vi "影像辨識-2.vi"() -> ()   [LabVIEW 2014]
uses:
  <vilib>/vision/NI_Vision_Development_Module.lvlib
panel:
  out "Image Pixels (U32) 3":u32[][](array[numeric])
  out "Image Pixels (U32) 2":u32[][](array[numeric])
  out "Image Pixels (U32)":u32[][](array[numeric])
  out "Pixel Value (U8)":u8
  out "Pixel Value (U32)":u32
  out "lumi 2":T1(plugin-control)
  out "saturastion":T1(plugin-control)
  in  "Stop (F)":bool
  out "Image Out":T1(plugin-control)
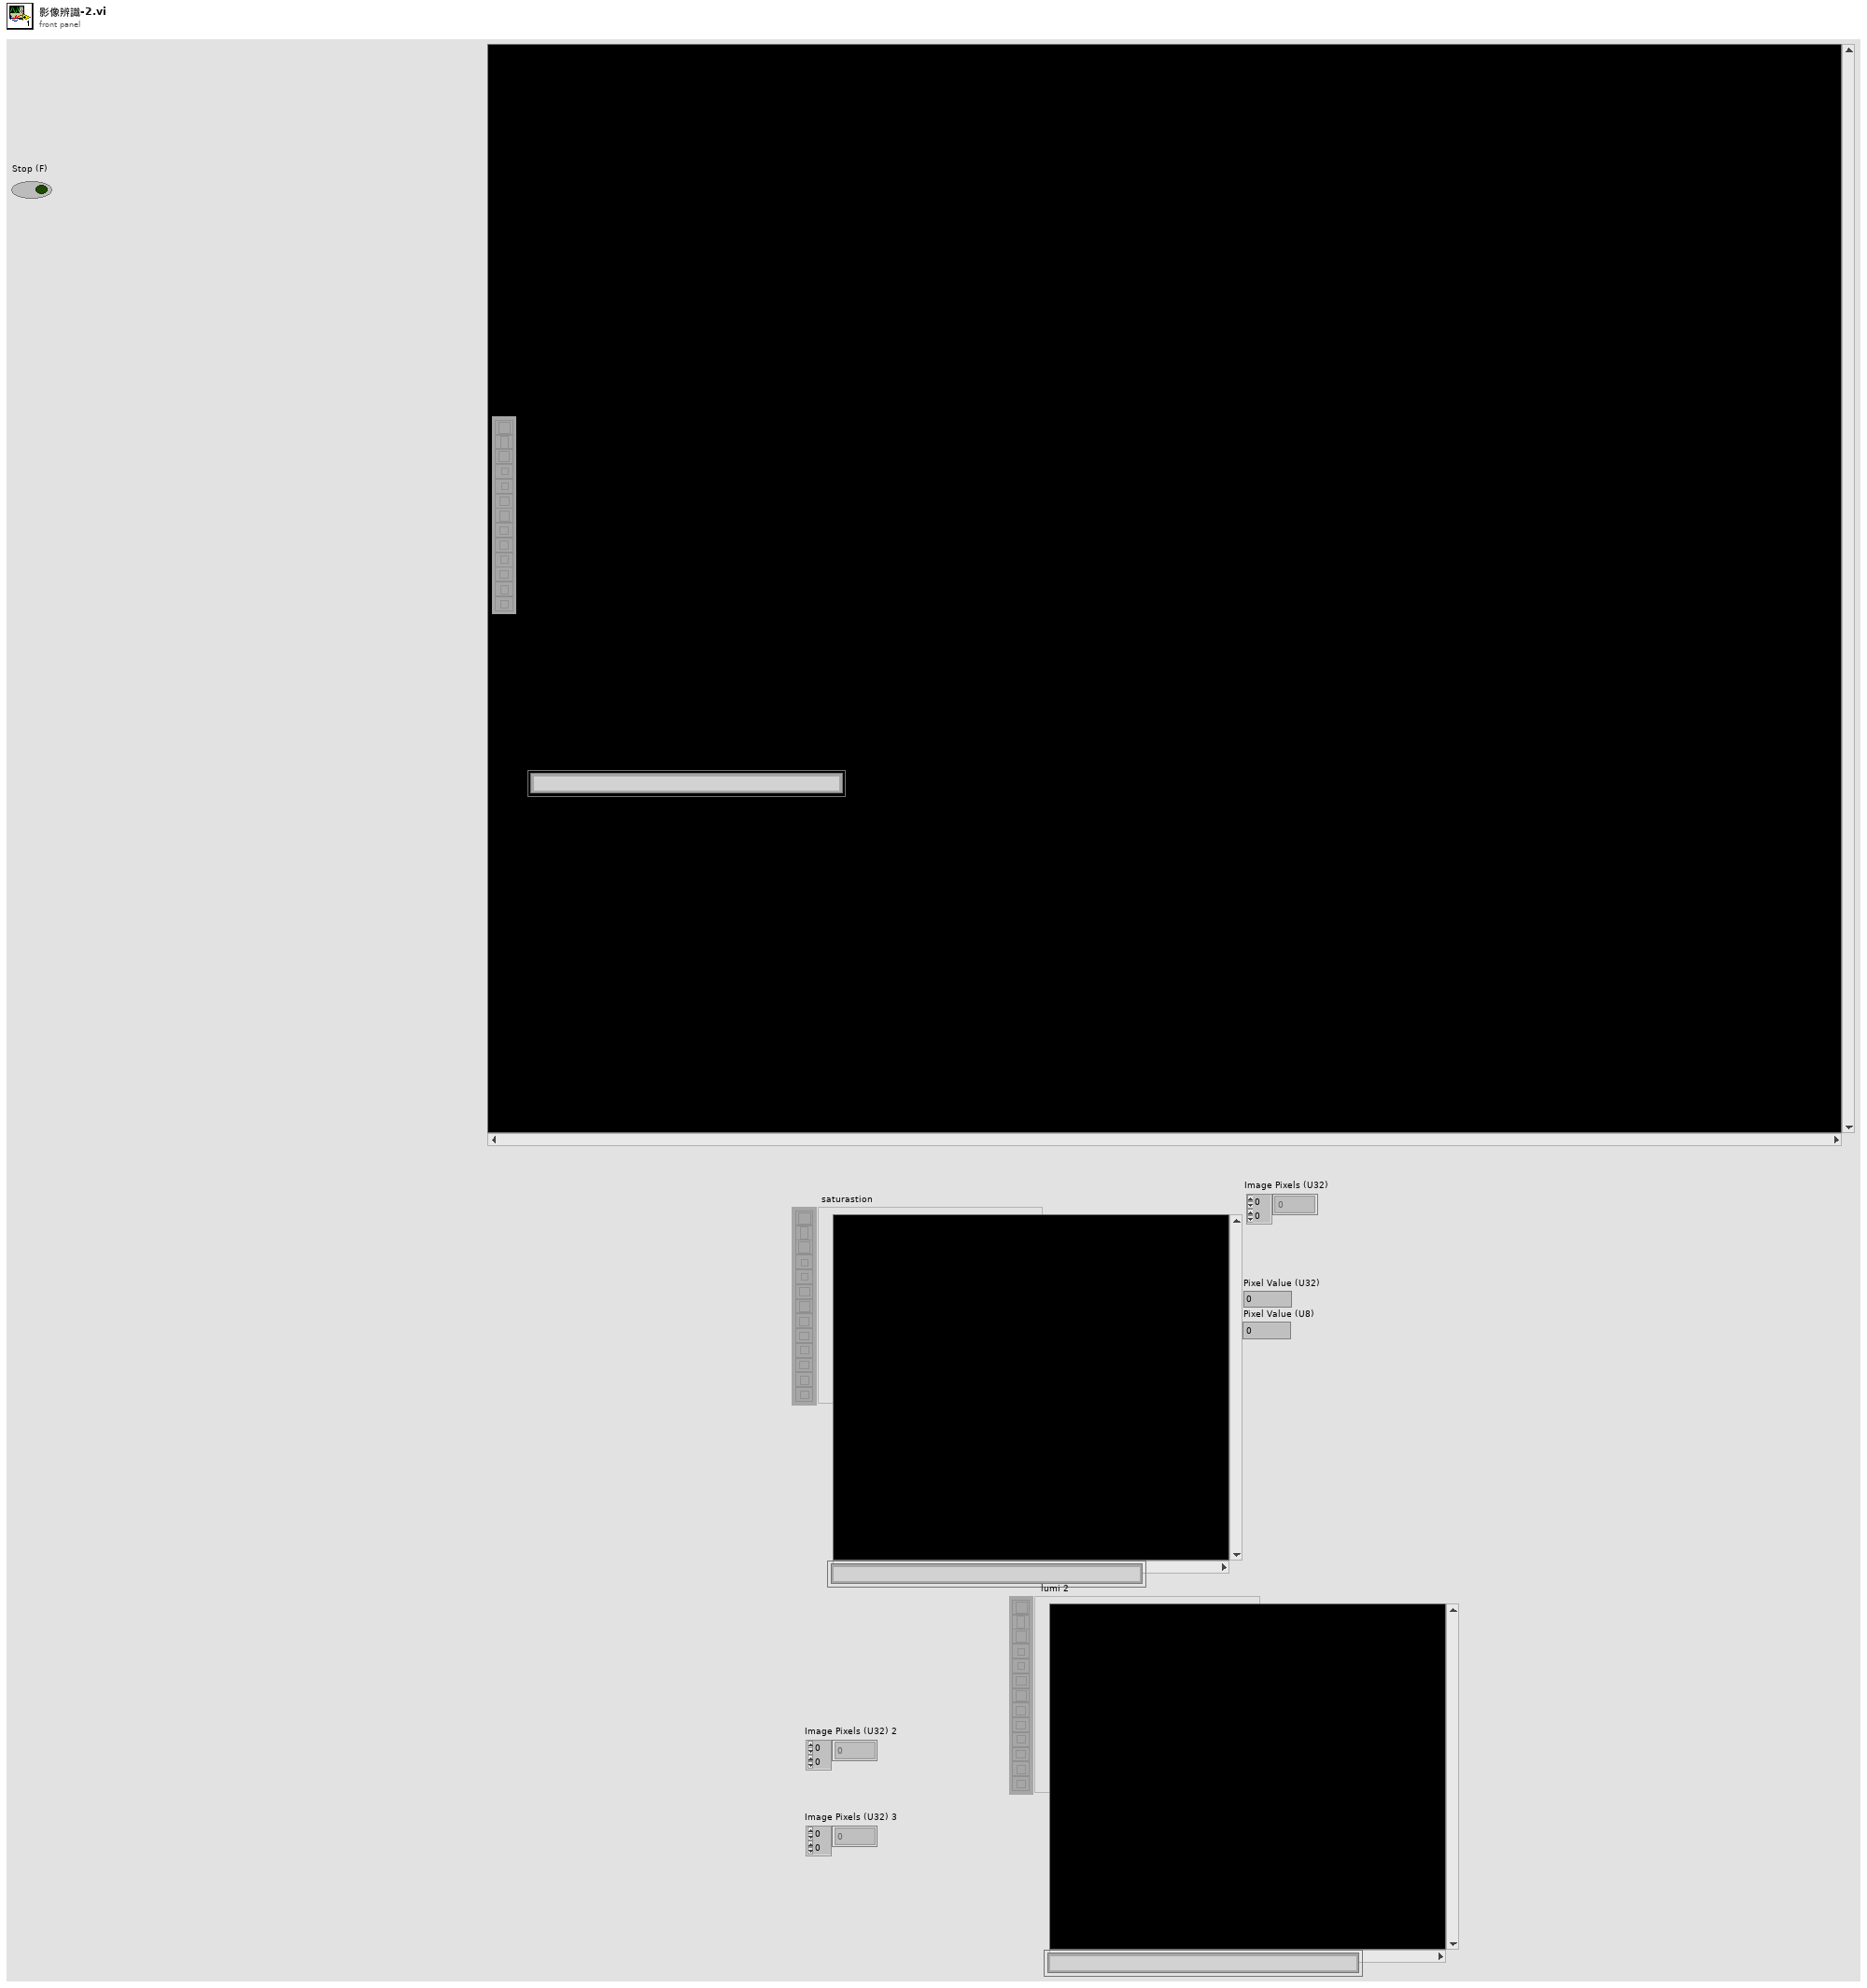
[diagram p1: front panel]
types:
  T1 = typedef "IMAQ Image.ctl" = refnum<image>
  T2 = typedef "Image Type" = u32
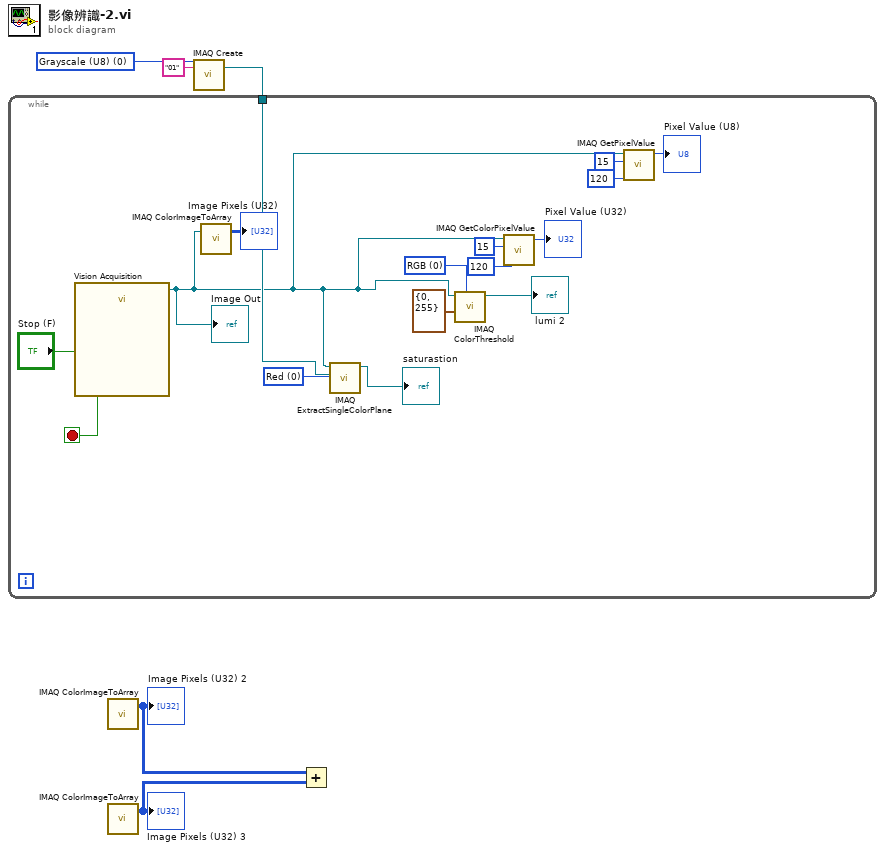
[diagram p0: block diagram]
diagram:
  w3 = T2 0 items=["Grayscale (U8)", "Grayscale (I16)", "Grayscale (SGL)", "Complex (CSG)", "RGB (U32)", "HSL (U32)", "RGB (U64)", "Grayscale (U16)"] ("Image Type")
  n1 = call "IMAQ ColorImageToArray"() -> ("Image Pixels (U32)"=w2:u32[][])  [unwired: 4 in, 2 out]
  "Image Pixels (U32) 2" <- w2
  n2 = call "IMAQ ColorImageToArray"() -> ("Image Pixels (U32)"=w1:u32[][])  [unwired: 4 in, 2 out]
  "Image Pixels (U32) 3" <- w1
  n3 = call "IMAQ Create"("Image Name"="01", "Image Type"=w3) -> ("New Image"=w5:T1)  [unwired: 3 in, 1 out]
  n4 = while {
    tunnel: w5 -> [w17]
    stop <- w20 stop-if-true
    w16 = u16 0 items=["RGB", "HSL", "HSV", "HSI"] ("Color Mode")
    w19 = 0 items=["Red", "Green", "Blue", "Hue", "Saturation", "Luminance", "Value", "Intensity"] ("Color Plane")
    n5 = call "Vision Acquisition"("Stop (F)"="Stop (F)") -> ("Image Out"=w7:T1, "Stopped"=w20:bool)  [unwired: 24 in, 1 out]
    "Image Out" <- w7
    n6 = call "IMAQ ColorImageToArray"("Image"=w7) -> ("Image Pixels (U32)"=→"Image Pixels (U32)":u32[][])  [unwired: 3 in, 2 out]
    n7 = call "IMAQ ExtractSingleColorPlane"("Color Plane"=w19, "Image Dst"=w17, "Image Src"=w7) -> ("Image Dst Out"=→"saturastion":T1)  [unwired: 7 in, 1 out]
    n8 = call "IMAQ ColorThreshold"("Color Mode"=w16, "Red or Hue Range"=cluster{"Lower value":i32, "Upper value":i32} {"Lower value"=0, "Upper value"=255}, "Image Src"=w7) -> ("Image Dst Out"=→"lumi 2":T1)  [unwired: 7 in, 1 out]
    n9 = call "IMAQ GetColorPixelValue"("Y Coordinate"=120, "X Coordinate"=15, "Image"=w7) -> ("Pixel Value (U32)"=→"Pixel Value (U32)":u32)  [unwired: 1 in, 2 out]
    n10 = call "IMAQ GetPixelValue"("Image"=w7, "X Coordinate"=15, "Y Coordinate"=120) -> ("Pixel Value (U8)"=→"Pixel Value (U8)":u8)  [unwired: 3 in, 4 out]
  }
  n11 = Add(x=w2, y=w1) -> ()  [unwired: 1 out]
